vi "BUILD_install and upload core.vi"(6 "Buildlog":path, 8 "error in":errorcluster, 9 "args":string[](array[string]), 11 "vip built path":path) -> (0 "error out":errorcluster)   [LabVIEW 2013]
uses:
  <vilib>/JKI/VIPM API/VIPM API_vipm_api.lvlib
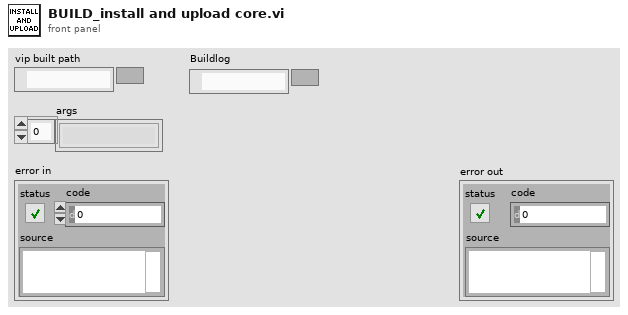
[diagram p1: front panel]
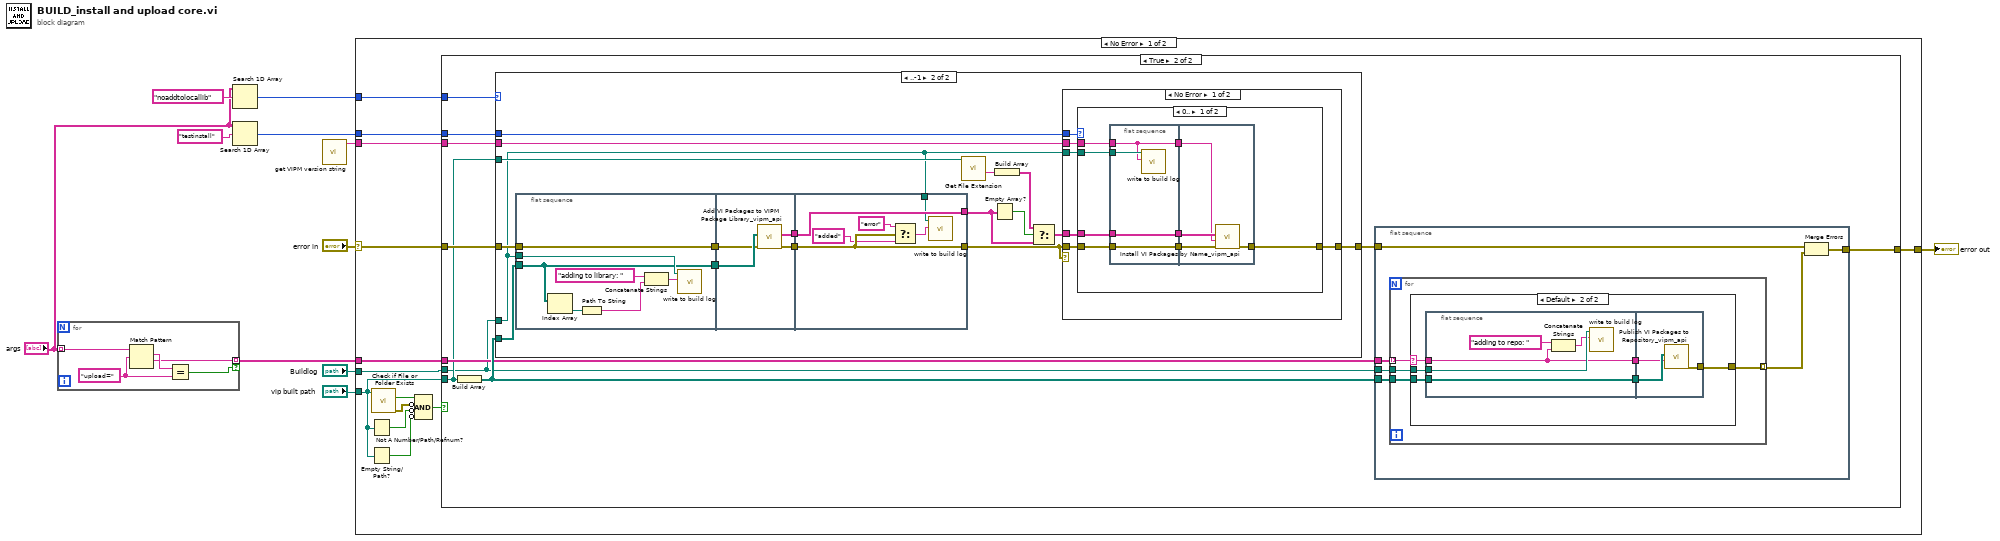
[diagram p0: block diagram]
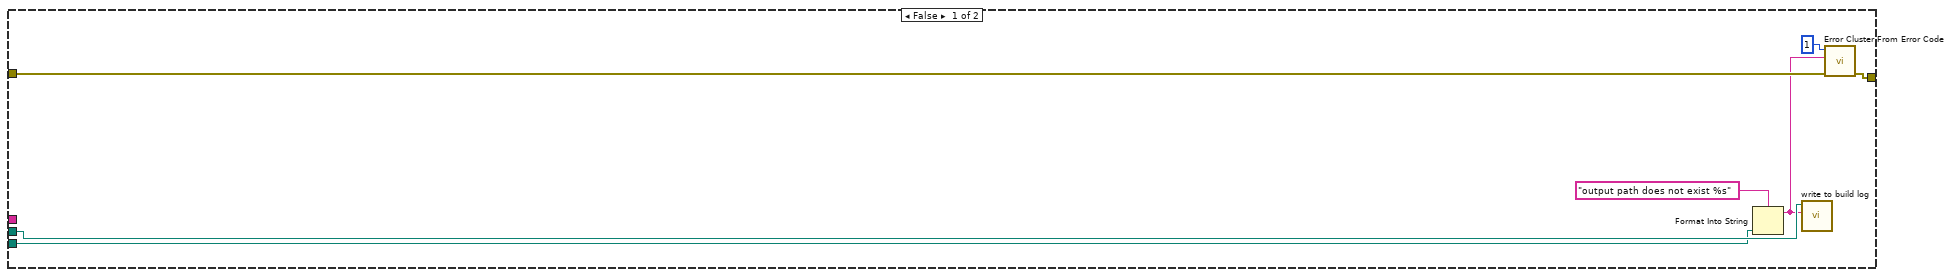
[diagram p2: hidden frame]
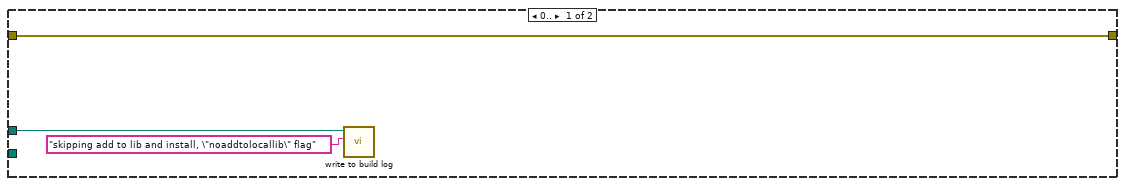
[diagram p3: hidden frame]
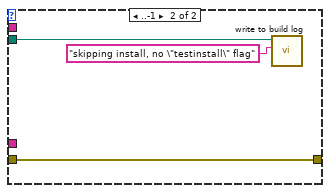
[diagram p4: hidden frame]
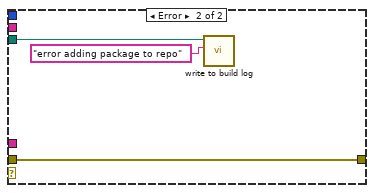
[diagram p5: hidden frame]
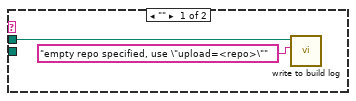
[diagram p6: hidden frame]
diagram:
  n1 = for {
    tunnel: "args" -> [w16] mode=indexing
    tunnel: [w13] -> w4 mode=indexing if=w12
    w14 = "upload=" ("regular expression")
    n2 = Match Pattern(string=w16, regular expression=w14) -> (match substring=w15:string, after substring=w13:string)  [unwired: 1 in, 2 out]
    n3 = Equal?(x=w15, y=w14) -> (x = y?=w12:bool)
  }
  n4 = Search 1D Array(1D array="args", element="noaddtolocallib") -> (index of element=w1:i32)  [unwired: 1 in]
  n5 = Search 1D Array(1D array="args", element="testinstall") -> (index of element=w5:i32)  [unwired: 1 in]
  n6 = call "get VIPM version string.vi"() -> ("version string"=w8:string)  [unwired: 11 in]
  n7 = case shown="No Error" "error in" {
    selector: "error in" -> [w27 w138]
    tunnel: "vip built path" -> [w19 _]
    tunnel: w8 -> [w29 _]
    tunnel: [w28 w138] -> w10
    tunnel: "Buildlog" -> [w26 _]
    tunnel: w5 -> [w25 _]
    tunnel: w4 -> [w24 _]
    tunnel: w1 -> [w17 _]
    frame No Error {
      n8 = Not A Number/Path/Refnum?(number/path/refnum=w19) -> (NaN/Path/Refnum?=w21:bool)
      n9 = Empty String/Path?(string/path=w19) -> (empty?=w20:bool)
      n10 = call <vilib>:"Check if File or Folder Exists.vi"("path"=w19) -> ("error out"=w22:errorcluster, "file or folder exists?"=w23:bool)  [unwired: 8 in, 1 out]
      n11 = Compound Arithmetic op=AND(w23, invert w22, invert w21, invert w20) -> (w18:bool)
      n12 = case shown="True" w18 {
        tunnel: w19 -> [w34 w39]
        tunnel: [w32 w45] -> w28
        tunnel: w29 -> [_ w44]
        tunnel: w27 -> [w36 w42]
        tunnel: w26 -> [w35 w38]
        tunnel: w25 -> [_ w41]
        tunnel: w24 -> [_ w40]
        tunnel: w17 -> [_ w37]
        frame False {
          n13 = Format Into String(format string="output path does not exist %s", w34) -> (resulting string=w30:string)  [unwired: 2 in, 1 out]
          n14 = call "write to build log.vi"("text"=w30, "log"=w35) -> ()  [unwired: 10 in]
          n15 = call <vilib>:"Error Cluster From Error Code.vi"("error in (no error)"=w36, "error message (\"\")"=w30, "error code (0)"=1) -> ("error out"=w32:errorcluster)  [unwired: 6 in]
        }
        frame True {
          n16 = Build Array(w39) -> (w46:path[])
          n17 = case shown="..-1" w37 {
            tunnel: w46 -> [_ w62]
            tunnel: w44 -> [_ w61]
            tunnel: [w47 w60] -> w43
            tunnel: w42 -> [w47 w53]
            tunnel: w41 -> [_ w52]
            tunnel: w39 -> [_ w51]
            tunnel: w38 -> [w48 w50]
            frame 0.. {
              n18 = call "write to build log.vi"("text"="skipping add to lib and install, \"noaddtolocallib\" flag", "log"=w48) -> ()  [unwired: 10 in]
            }
            frame ..-1 {
              n19 = flat-sequence {
                tunnel: w53 -> [w73]
                tunnel: w62 -> [w67]
                tunnel: [w67] -> w66
                tunnel: [w73] -> w65
                tunnel: w50 -> [w72]
                tunnel: [w76] -> w64
                tunnel: [w75] -> w63
                tunnel: w66 -> [w77]
                tunnel: w65 -> [w74]
                tunnel: [w83] -> w57
                tunnel: [w82] -> w59
                tunnel: w64 -> [w82]
                tunnel: w63 -> [w83]
                tunnel: w50 -> [w78]
                frame #0 {
                  n20 = Index Array(array=w67) -> (element=w68:path)  [unwired: 1 in]
                  n21 = Path To String(path=w68) -> (string=w69:string)
                  n22 = Concatenate Strings("adding to library: " ("string"), w69) -> (w70:string)
                  n23 = call "write to build log.vi"("text"=w70, "log"=w72) -> ()  [unwired: 10 in]
                }
                frame #1 {
                  n24 = call <vilib>:"Add VI Packages to VIPM Package Library_vipm_api.vi"("error in (no error)"=w74, "Packages to add to VIPM Library (vipc,vip,ogp)"=w77) -> ("error out"=w76:errorcluster, "Package Names Added"=w75:string[])  [unwired: 8 in]
                }
                frame #2 {
                  n25 = Select(t="error" ("string"), s=w82, f="added" ("string")) -> (s? t:f=w79:string)
                  n26 = call "write to build log.vi"("text"=w79, "log"=w78) -> ()  [unwired: 10 in]
                }
              }
              n27 = call <vilib>:"Get File Extension.vi"("file"=w51) -> ("filename without extension"=w55:string)  [unwired: 7 in, 3 out]
              n28 = Empty Array?(array=w57) -> (empty?=w58:bool)
              n29 = Build Array(w55) -> (w54:string[])
              n30 = Select(t=w54, s=w58, f=w57) -> (s? t:f=w56:string[])
              n31 = case shown="No Error" w59 {
                tunnel: w59 -> [w89 w111]
                tunnel: w56 -> [w88 _]
                tunnel: w61 -> [w87 _]
                tunnel: [w86 w111] -> w60
                tunnel: w50 -> [w84 w110]
                tunnel: w52 -> [w85 _]
                frame No Error {
                  n32 = case shown="0.." w85 {
                    tunnel: w89 -> [w97 w108]
                    tunnel: w88 -> [w96 _]
                    tunnel: w87 -> [w95 _]
                    tunnel: [w94 w108] -> w86
                    tunnel: w84 -> [w90 w107]
                    frame 0.. {
                      n33 = flat-sequence {
                        tunnel: w95 -> [w98]
                        tunnel: w96 -> [w100]
                        tunnel: w97 -> [w101]
                        tunnel: [w101] -> w93
                        tunnel: [w100] -> w92
                        tunnel: [w98] -> w91
                        tunnel: w90 -> [w99]
                        tunnel: [w102] -> w94
                        tunnel: w93 -> [w105]
                        tunnel: w92 -> [w104]
                        tunnel: w91 -> [w103]
                        frame #0 {
                          n34 = call "write to build log.vi"("text"=w98, "log"=w99) -> ()  [unwired: 10 in]
                        }
                        frame #1 {
                          n35 = call <vilib>:"Install VI Packages by Name_vipm_api.vi"("error in (no error)"=w105, "LabVIEW Version"=w103, "Package Names to Install []"=w104) -> ("error out"=w102:errorcluster)  [unwired: 8 in]
                        }
                      }
                    }
                    frame ..-1 {
                      n36 = call "write to build log.vi"("text"="skipping install, no \"testinstall\" flag", "log"=w107) -> ()  [unwired: 10 in]
                    }
                  }
                }
                frame Error {
                  n37 = call "write to build log.vi"("text"="error adding package to repo", "log"=w110) -> ()  [unwired: 10 in]
                }
              }
            }
          }
          n38 = flat-sequence {
            tunnel: w46 -> [w117]
            tunnel: [w116] -> w45
            tunnel: w43 -> [w112]
            tunnel: w40 -> [w115]
            tunnel: w38 -> [w114]
            frame #0 {
              n39 = for {
                tunnel: w117 -> [w121]
                tunnel: [w120] -> w113 mode=indexing
                tunnel: w115 -> [w119] mode=indexing
                tunnel: w114 -> [w118]
                n40 = case shown="Default" w119 {
                  selector: w119 -> [_ w127]
                  tunnel: w121 -> [_ w129]
                  tunnel: [_ w128] -> w120
                  tunnel: w118 -> [w123 w124]
                  frame "" {
                    n41 = call "write to build log.vi"("text"="empty repo specified, use \"upload=<repo>\"", "log"=w123) -> ()  [unwired: 10 in]
                  }
                  frame Default {
                    n42 = flat-sequence {
                      tunnel: w127 -> [w131]
                      tunnel: w129 -> [w134]
                      tunnel: [w134] -> w126
                      tunnel: [w131] -> w125
                      tunnel: w124 -> [w133]
                      tunnel: [w136] -> w128
                      tunnel: w126 -> [w137]
                      tunnel: w125 -> [w135]
                      frame #0 {
                        n43 = Concatenate Strings("adding to repo: " ("string"), w131) -> (w132:string)
                        n44 = call "write to build log.vi"("text"=w132, "log"=w133) -> ()  [unwired: 10 in]
                      }
                      frame #1 {
                        n45 = call <vilib>:"Publish VI Packages to Repository_vipm_api.vi"("Repository Name"=w135, "Packages to publish to Repository Library (vip,ogp)"=w137) -> ("error out"=w136:errorcluster)  [unwired: 8 in, 1 out]
                      }
                    }
                  }
                }
              }
              n46 = Merge Errors(w112, w113) -> (w116:errorcluster)
            }
          }
        }
      }
    }
    frame Error {
    }
  }
  "error out" <- w10
